vi "execute_initial_value_policy.vi"(8 "error in (no error)":errorcluster, 9 "Last Publish Time":timestamp, 10 "Last Topic Value":variant, 11 "OneShotSubscription In":refnum<class "OneShotSubscription.lvclass">) -> (0 "error out":errorcluster, 3 "OneShotSubscription Out":refnum<class "OneShotSubscription.lvclass">)   [LabVIEW 2015, in "SubscriptionPolicy.lvlib" / "OneShotSubscription.lvclass"]
uses:
  OneShotSubscription.lvclass
  OneShotSubscription.lvclass/OneShotSubscription.ctl
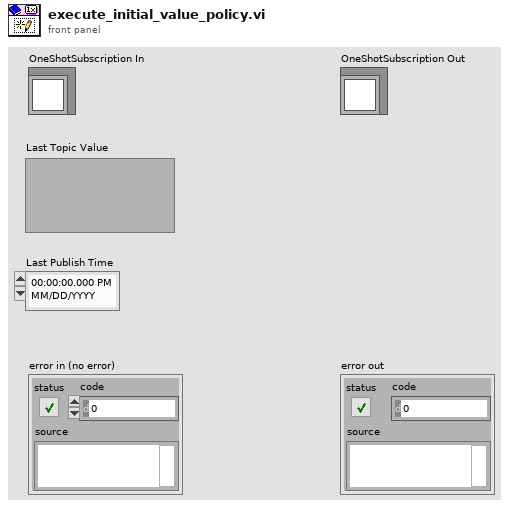
[diagram p1: front panel]
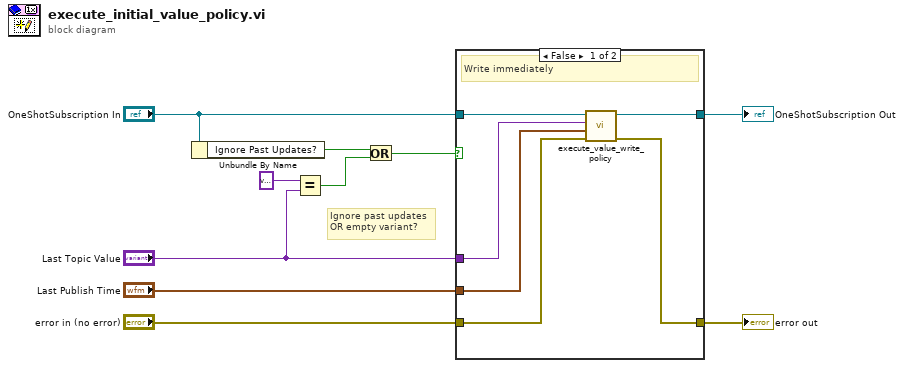
[diagram p0: block diagram]
diagram:
  # "Ignore past updates\nOR empty variant?"
  n1 = Unbundle By Name("OneShotSubscription In") -> ("Ignore Past Updates?"=w9:bool)
  n2 = Equal?(x=variant, y="Last Topic Value") -> (x = y?=w8:bool)
  n3 = Or(x=w9, y=w8) -> (x .or. y?=w7:bool)
  n4 = case shown="False" w7 {
    tunnel: "OneShotSubscription In" -> [w16 w18]
    tunnel: [w15 w18] -> w6
    tunnel: "Last Topic Value" -> [w11 _]
    tunnel: "Last Publish Time" -> [w13 _]
    tunnel: "error in (no error)" -> [w14 w17]
    tunnel: [w12 w17] -> w3
    frame False {
      # "Write immediately"
      n5 = call-dynamic "execute_value_write_policy.vi"("error in (no error)"=w14, "Publish Time"=w13, "New Topic Value"=w11, "OneShotSubscription In"=w16) -> ("error out"=w12:errorcluster, "OneShotSubscription Out"=w15:refnum<class "OneShotSubscription.lvclass">)  [unwired: 6 in]
    }
    frame True {
      # "Do not write immediately"
    }
  }
  "error out" <- w3
  "OneShotSubscription Out" <- w6
